vi "Master with follower.vi"   [LabVIEW 2016, in "Moving Motor.lvrbt"]
uses:
  Moving Motor.lvrbt
  <vilib>/NXT/Block Support/NXT_InputPort.ctl
  <vilib>/NXT/Hardware/Plugins/Tetrix DC Motor/TetrixDCMotorAddress.ctl
  <vilib>/NXT/NXTIO Xnodes/NXTIONodeSubVIs/TETRIX IO Move DC Motors.vi
  <vilib>/NXT/Dual Mode Library/Sensors/EV3_Color_Color.vi
  <vilib>/NXT/NXTIO Xnodes/NXTIONodeSubVIs/TETRIX IO Stop DC Motors.vi
  <vilib>/NXT/Dual Mode Library/Waits/Wait_Num.vi
  <vilib>/NXT/Dual Mode Library/Sensors/EV3_Color_Reflect.vi
  <vilib>/NXT/Subs/LVHSConnector.ctl
  <vilib>/NXT/NXTIO Xnodes/AddressXNode/NXTIOAddress.xnode
  <vilib>/NXT/NXTIO Xnodes/NXTIOXNode/NXTIO.xnode
  <vilib>/NXT/LegoClasses/BrickReference/BrickReference.lvclass
types:
  T1 = typedef "TetrixDCMotorAddress.ctl" = i32
  T2 = typedef "LVHSConnector.ctl" = refnum<class "BrickReference.lvclass">
  T3 = cluster{"TetrixDCMotor":T1, "TetrixDCMotor 2":T1}
  T4 = typedef "NXT_InputPort.ctl" = u32
  T5 = typedef "ColorSensorColors.ctl" = enum16{"No Color", "Black", "Blue", "Green", "Yellow", "Red", "White", "Brown"}
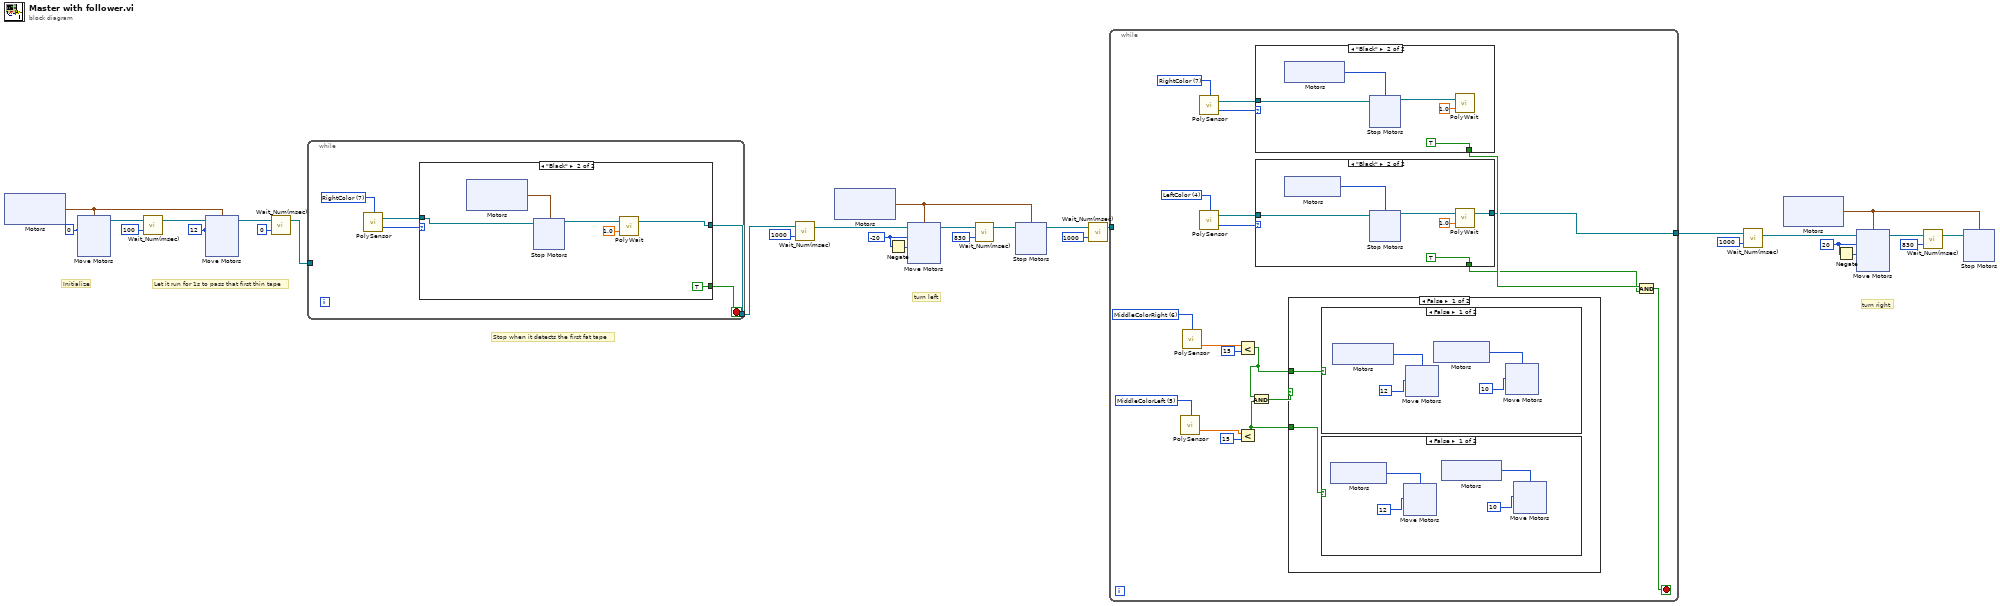
[diagram p0: block diagram]
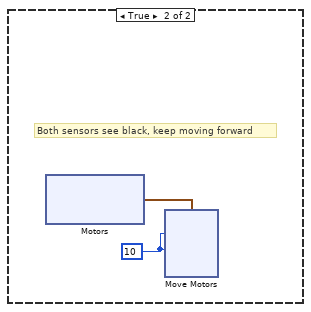
[diagram p4: hidden frame]
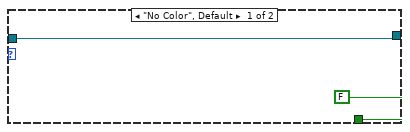
[diagram p5: hidden frame]
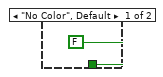
[diagram p6: hidden frame]
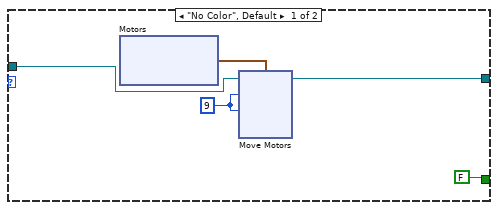
[diagram p7: hidden frame]
diagram:
  w6 = i8 20 ("Power/Speed 1")
  w17 = i8 -20 ("Power/Speed 1")
  w14 = i8 12 ("Power/Speed 1")
  w30 = i8 0 ("Power/Speed 1")
  # "turn right"
  # "turn left"
  # "Stop when it detects the first fat tape"
  # "Let it run for 1s to pass that first thin tape"
  # "Initialize"
  n1 = xnode "Motors"() -> ("Motor"=w24:cluster{"TetrixDCMotor":T1, "TetrixDCMotor":T1})
  n2 = xnode "Move Motors"("Power/Speed 2"=w30, "Power/Speed 1"=w30, "Motors"=w24) -> ("NXT/EV3"=w29:T2)  [unwired: 1 in]
  n3 = call <vilib>:"Wait_Num(msec).vi"("Time (100 msec)"=u32 100, "NXT/EV3"=w29) -> ("NXT/EV3"=w25:T2)  [unwired: 2 in]
  n4 = xnode "Move Motors"("Power/Speed 2"=w14, "Power/Speed 1"=w14, "Motors"=w24, "NXT/EV3"=w25) -> ("NXT/EV3"=w27:T2)
  n5 = call <vilib>:"Wait_Num(msec).vi"("Time (100 msec)"=u32 0, "NXT/EV3"=w27) -> ("NXT/EV3"=w23:T2)  [unwired: 2 in]
  n6 = while {
    tunnel: w23 -> [_]
    tunnel: [w33] -> w1
    stop <- w31 stop-if-true
    w35 = T4 7 items=["Port 1"=0, "Port 2"=1, "Port 3"=2, "Port 4"=3, "LeftColor"=4, "RightColor"=7] ("Port (Port 1)")
    n7 = call-poly <vilib>:"PolySensor.vi"("Port (Port 1)"=w35) -> ("Detected Color"=w34:T5, "NXT/EV3"=w32:T2)  [unwired: 2 in]
    n8 = case shown="\"Black\"" w34 {
      tunnel: [FALSE TRUE] -> w31
      tunnel: [w37 w51] -> w33
      tunnel: w32 -> [w36 w50]
      frame "No Color", Default {
        w39 = i8 9 ("Power/Speed 1")
        n9 = xnode "Motors"() -> ("Motor"=w40:cluster{"TetrixDCMotor":T1, "TetrixDCMotor":T1})
        n10 = xnode "Move Motors"("Power/Speed 2"=w39, "Power/Speed 1"=w39, "Motors"=w40, "NXT/EV3"=w36) -> ("NXT/EV3"=w37:T2)
      }
      frame "Black" {
        n11 = xnode "Motors"() -> ("Motor"=w55:cluster{"TetrixDCMotor":T1, "TetrixDCMotor":T1})
        n12 = xnode "Stop Motors"("Motors"=w55, "NXT/EV3"=w50) -> ("NXT/EV3"=w53:T2)
        n13 = call-poly <vilib>:"PolyWait.vi"("Time (1 sec)"=sgl 1.0, "NXT/EV3"=w53) -> ("NXT/EV3"=w51:T2)  [unwired: 2 in]
      }
    }
  }
  n14 = call <vilib>:"Wait_Num(msec).vi"("Time (100 msec)"=u32 1000, "NXT/EV3"=w1) -> ("NXT/EV3"=w15:T2)  [unwired: 2 in]
  n15 = xnode "Motors"() -> ("Motor"=w19:cluster{"TetrixDCMotor":T1, "TetrixDCMotor":T1})
  n16 = Negate(x=w17) -> (-x=w18:i8)
  n17 = xnode "Move Motors"("Power/Speed 2"=w18, "Power/Speed 1"=w17, "Motors"=w19, "NXT/EV3"=w15) -> ("NXT/EV3"=w22:T2)
  n18 = call <vilib>:"Wait_Num(msec).vi"("Time (100 msec)"=u32 830, "NXT/EV3"=w22) -> ("NXT/EV3"=w20:T2)  [unwired: 2 in]
  n19 = xnode "Stop Motors"("Motors"=w19, "NXT/EV3"=w20) -> ("NXT/EV3"=w12:T2)
  n20 = call <vilib>:"Wait_Num(msec).vi"("Time (100 msec)"=u32 1000, "NXT/EV3"=w12) -> ("NXT/EV3"=w3:T2)  [unwired: 2 in]
  n21 = while {
    tunnel: w3 -> [_]
    tunnel: [w62] -> w2
    stop <- w63 stop-if-true
    w71 = T4 5 items=["MiddleColorLeft"=5, "Port 1"=0, "Port 2"=1, "Port 3"=2, "Port 4"=3] ("ColorLeft")
    w72 = T4 6 items=["Port 1"=0, "Port 2"=1, "Port 3"=2, "Port 4"=3, "MiddleColorRight"=6] ("ColorRight")
    w77 = T4 4 items=["Port 1"=0, "Port 2"=1, "Port 3"=2, "Port 4"=3, "LeftColor"=4, "RightColor"=7] ("Port (Port 1)")
    w80 = T4 7 items=["Port 1"=0, "Port 2"=1, "Port 3"=2, "Port 4"=3, "LeftColor"=4, "RightColor"=7] ("Port (Port 1)")
    n22 = call-poly <vilib>:"PolySensor.vi"("Port (Port 1)"=w71) -> ("Scaled Value"=w67:sgl)  [unwired: 2 in, 1 out]
    n23 = call-poly <vilib>:"PolySensor.vi"("Port (Port 1)"=w72) -> ("Scaled Value"=w70:sgl)  [unwired: 2 in, 1 out]
    n24 = call-poly <vilib>:"PolySensor.vi"("Port (Port 1)"=w80) -> ("Detected Color"=w79:T5, "NXT/EV3"=w78:T2)  [unwired: 2 in]
    n25 = call-poly <vilib>:"PolySensor.vi"("Port (Port 1)"=w77) -> ("Detected Color"=w76:T5, "NXT/EV3"=w75:T2)  [unwired: 2 in]
    n26 = Less?(x=w70, y=i16 15) -> (x < y?=w65:bool)
    n27 = Less?(x=w67, y=i16 15) -> (x < y?=w64:bool)
    n28 = And(x=w65, y=w64) -> (x .and. y?=w66:bool)
    n29 = case shown="\"Black\"" w79 {
      tunnel: [FALSE TRUE] -> w74
      tunnel: w78 -> [_ w149]
      frame "No Color", Default {
      }
      frame "Black" {
        n30 = xnode "Motors"() -> ("Motor"=w153:T1)
        n31 = xnode "Stop Motors"("Motors"=w153, "NXT/EV3"=w149) -> ("NXT/EV3"=w151:T2)
        n32 = call-poly <vilib>:"PolyWait.vi"("Time (1 sec)"=sgl 1.0, "NXT/EV3"=w151) -> ()  [unwired: 2 in, 1 out]
      }
    }
    n33 = case shown="\"Black\"" w76 {
      tunnel: [FALSE TRUE] -> w73
      tunnel: w75 -> [w134 w137]
      tunnel: [w134 w136] -> w62
      frame "No Color", Default {
      }
      frame "Black" {
        n34 = xnode "Motors"() -> ("Motor"=w141:T1)
        n35 = xnode "Stop Motors"("Motors"=w141, "NXT/EV3"=w137) -> ("NXT/EV3"=w139:T2)
        n36 = call-poly <vilib>:"PolyWait.vi"("Time (1 sec)"=sgl 1.0, "NXT/EV3"=w139) -> ("NXT/EV3"=w136:T2)  [unwired: 2 in]
      }
    }
    n37 = case "Case 1 and 4" shown="False" w66 {
      tunnel: w65 -> [w82 _]
      tunnel: w64 -> [w81 _]
      frame False {
        n38 = case shown="False" w82 {
          frame False {
            n39 = xnode "Motors"() -> ("Motor"=w105:T1)
            n40 = xnode "Move Motors"("Power/Speed 1"=i8 12 ("Power/Speed 2"), "Motors"=w105) -> ()  [unwired: 1 in, 1 out]
            n41 = xnode "Motors"() -> ("Motor"=w103:T1)
            n42 = xnode "Move Motors"("Power/Speed 1"=i8 10 ("Power/Speed 2"), "Motors"=w103) -> ()  [unwired: 1 in, 1 out]
          }
          frame True {
          }
        }
        n43 = case shown="False" w81 {
          frame False {
            n44 = xnode "Motors"() -> ("Motor"=w86:T1)
            n45 = xnode "Move Motors"("Power/Speed 1"=i8 12 ("Power/Speed 2"), "Motors"=w86) -> ()  [unwired: 1 in, 1 out]
            n46 = xnode "Motors"() -> ("Motor"=w84:T1)
            n47 = xnode "Move Motors"("Power/Speed 1"=i8 10 ("Power/Speed 2"), "Motors"=w84) -> ()  [unwired: 1 in, 1 out]
          }
          frame True {
          }
        }
      }
      frame True {
        w123 = i8 10 ("Power/Speed 2")
        # "Both sensors see black, keep moving forward"
        n48 = xnode "Motors"() -> ("Motor"=w124:cluster{"TetrixDCMotor":T1, "TetrixDCMotor":T1})
        n49 = xnode "Move Motors"("Power/Speed 2"=w123, "Power/Speed 1"=w123, "Motors"=w124) -> ()  [unwired: 1 in, 1 out]
      }
    }
    n50 = And(x=w74, y=w73) -> (x .and. y?=w63:bool)
  }
  n51 = call <vilib>:"Wait_Num(msec).vi"("Time (100 msec)"=u32 1000, "NXT/EV3"=w2) -> ("NXT/EV3"=w4:T2)  [unwired: 2 in]
  n52 = xnode "Motors"() -> ("Motor"=w8:cluster{"TetrixDCMotor":T1, "TetrixDCMotor":T1})
  n53 = Negate(x=w6) -> (-x=w7:i8)
  n54 = xnode "Move Motors"("Power/Speed 2"=w7, "Power/Speed 1"=w6, "Motors"=w8, "NXT/EV3"=w4) -> ("NXT/EV3"=w11:T2)
  n55 = call <vilib>:"Wait_Num(msec).vi"("Time (100 msec)"=u32 830, "NXT/EV3"=w11) -> ("NXT/EV3"=w9:T2)  [unwired: 2 in]
  n56 = xnode "Stop Motors"("Motors"=w8, "NXT/EV3"=w9) -> ()  [unwired: 1 out]
